vi "Flush and Clear.vi"(8 "error in (no error)":errorcluster, 11 "Sequencer Core in":refnum<class "Sequencer Core.lvclass">) -> (0 "error dub":errorcluster, 3 "Sequencer Core out":refnum<class "Sequencer Core.lvclass">)   [LabVIEW 2020, in "Sequencer.lvlib" / "Sequencer Core.lvclass"]
doc: "Flush the Sequencer Core and cancel any notification on the interrupt notifier."
uses:
  Sequencer Core.lvclass
  Sequencer Core.lvclass/Sequencer Core.ctl
  Message Priority Queue/Message Priority Queue.lvclass
  PPL/HDH.Data.Generic.lvlibp/Synchronization/Notifier/Notifier.lvclass
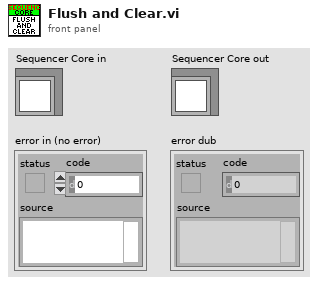
[diagram p1: front panel]
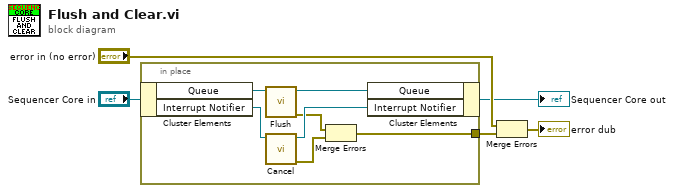
[diagram p0: block diagram]
diagram:
  n1 = in-place {
    in-place-border: [w6] -> w3
    n2 = in-place-cluster #1("Sequencer Core in") -> ("Queue"=w12:refnum<class "Message Priority Queue.lvclass">, "Interrupt Notifier"=w10:refnum<class "Notifier.lvclass">)
    n3 = call "Flush.vi"("Priority Queue in"=w12) -> ("error out"=w8:errorcluster, "Priority Queue out"=w11:refnum<class "Message Priority Queue.lvclass">)  [unwired: 8 in, 1 out]
    n4 = call "Cancel.vi"("Notifier in"=w10) -> ("error out"=w7:errorcluster, "Notifier out"=w9:refnum<class "Notifier.lvclass">)  [unwired: 8 in, 1 out]
    n5 = Merge Errors(w8, w7) -> (w6:errorcluster)
    n6 = in-place-cluster #1("Queue"=w11, "Interrupt Notifier"=w9) -> (→"Sequencer Core out":refnum<class "Sequencer Core.lvclass">)
  }
  n7 = Merge Errors("error in (no error)", w3) -> (→"error dub":errorcluster)
